vi "Micron Optics sm130 Triggered Acquisition.vi"() -> ()   [LabVIEW 2024]
doc: "Demonstrates the triggered peak wavelength acquisition. The peak wavelength acquisition can be untriggered, software or hardware triggered. \n\n<b>Note:</b>\nThis example is made for the instrument without channel multiplexer. Modifications will have to be made for instruments with channel multiplexer."
uses:
  Micron Optics sm130.lvlib
panel:
  in  "Trigger Type (0:Untriggered)":u16(ring) items=["Untriggered", "Software Triggered", "Hardware Triggered"]
  in  "Sensor Number (1)":i32=1
  in  "Channel (1: Channel 1)":i32(ring)=1 items=["Channel 1"=1, "Channel 2"=2, "Channel 3"=3, "Channel 4"=4]
  out "Peak Wavelength Chart":dbl(graph)
  in  "Stop":bool
  in  "Stop Trigger":bool
  in  "Start Trigger":bool
  in  "Data Interleave (1)":i32=1
  in  "Number of Acquisitions (100)":i32=100
  in  "Trigger Stop Condition (1:Edge Triggering)":u16(ring)=1 items=["Number of Acquisitions", "Edge Triggering"]
  in  "Trigger Stop Edge (0: Rising)":u16(ring) items=["Rising", "Falling"]
  in  "Trigger Start Edge (0: Rising)":u16(ring) items=["Rising", "Falling"]
  in  "VISA resource name":refnum<visa-resource-name>
  # "(c) 2009 - 2012 National Instruments.  ALL RIGHTS RESERVED."
  # "Sensor View"
  # "Trigger Control"
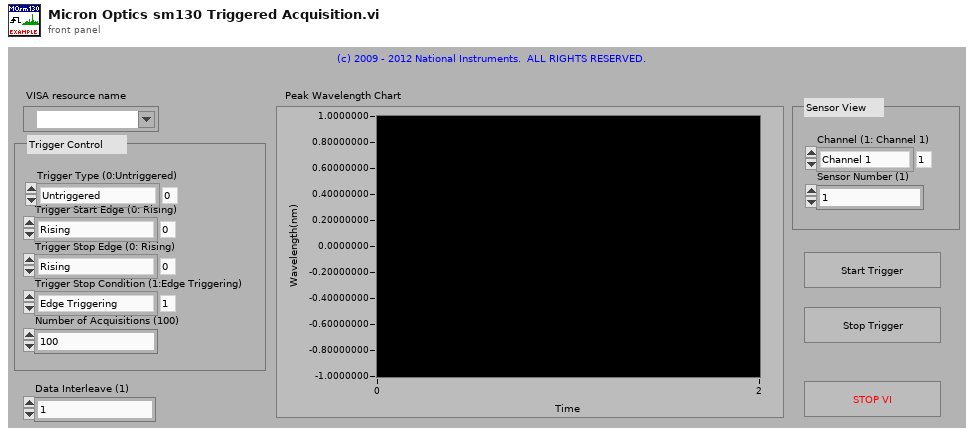
[diagram p1: front panel]
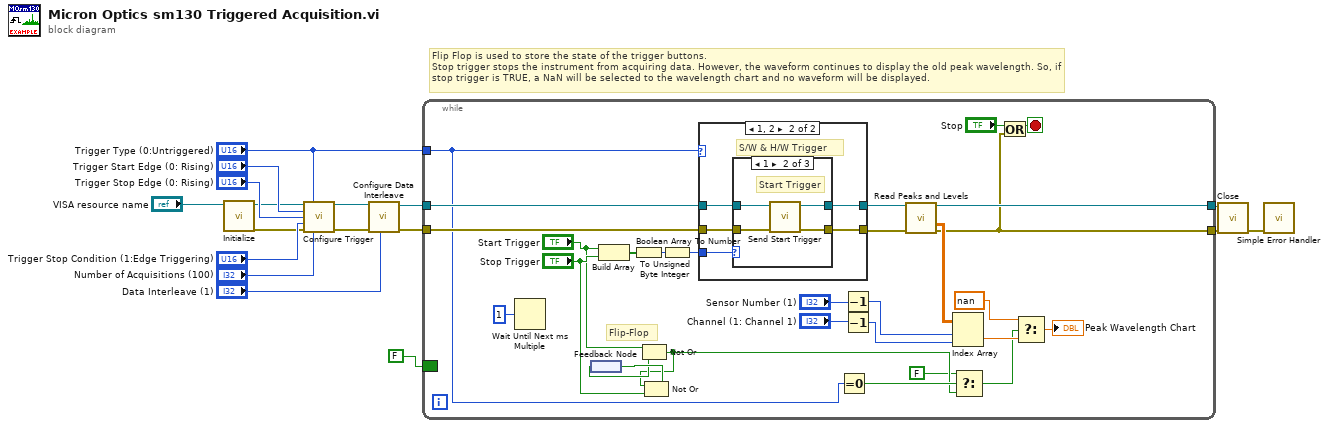
[diagram p0: block diagram]
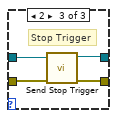
[diagram p4: hidden frame]
diagram:
  # "Flip Flop is used to store the state of the trigger buttons. \nStop trigger stops the instrument from acquiring data. However, the waveform continues to display the old peak wavelength. So, if stop trigger is TRUE, a NaN will be selected to the wavelength chart and no waveform will be displayed."
  n1 = call "Initialize.vi"("VISA resource name"="VISA resource name") -> ("error out"=w8:errorcluster, "VISA resource name out"=w9:refnum<visa-resource-name>)  [unwired: 9 in]
  n2 = call "Configure Trigger.vi"("VISA resource name"=w9, "Trigger Type (0:Untriggered)"="Trigger Type (0:Untriggered)", "Trigger Start Edge (0: Rising)"="Trigger Start Edge (0: Rising)", "Trigger Stop Edge (0: Rising)"="Trigger Stop Edge (0: Rising)", "Trigger Stop Condition (1:Edge Triggering)"="Trigger Stop Condition (1:Edge Triggering)", "error in (no error)"=w8, "Number of Acquisitions (100)"="Number of Acquisitions (100)") -> ("VISA resource name out"=w12:refnum<visa-resource-name>, "error out"=w11:errorcluster)  [unwired: 6 in, 1 out]
  n3 = call "Configure Data Interleave.vi"("Data Interleave (1)"="Data Interleave (1)", "error in (no error)"=w11, "VISA resource name"=w12) -> ("error out"=w5:errorcluster, "VISA resource name out"=w6:refnum<visa-resource-name>)  [unwired: 7 in]
  n4 = while {
    tunnel: w6 -> [w41]
    tunnel: w5 -> [w43]
    tunnel: "Trigger Type (0:Untriggered)" -> [w22]
    tunnel: [w26] -> w4
    tunnel: [w18] -> w3
    border: FALSE -> [_]
    stop <- w19 stop-if-true
    # "Flip-Flop"
    n5 = Wait Until Next ms Multiple(millisecond multiple=u32 1) -> ()  [unwired: 1 out]
    n6 = feedback #1() -> (w29:bool)
    n7 = Build Array("Start Trigger", "Stop Trigger") -> (w46:bool[])
    n8 = Boolean Array To Number(Boolean array=w46) -> (number=w45:u32)
    n9 = Not Or(1:w29, 2:"Start Trigger") -> (0:w23:bool)
    n10 = Not Or(1:"Stop Trigger", 2:w23) -> (0:w30:bool)
    n11 = feedback-in #1(w30) -> ()
    n12 = To Unsigned Byte Integer(number=w45) -> (unsigned 8bit integer=w44:u8)
    n13 = case shown="1, 2" w22 {
      tunnel: w44 -> [_ w53]
      tunnel: w41 -> [w48 w52]
      tunnel: w43 -> [w47 w51]
      tunnel: [w47 w50] -> w38
      tunnel: [w48 w49] -> w39
      frame 0, Default {
        # "Untriggered"
      }
      frame 1, 2 {
        # "S/W & H/W Trigger"
        n14 = case shown="1" w53 {
          tunnel: w52 -> [w55 w59 w63]
          tunnel: w51 -> [w54 w58 w60]
          tunnel: [w55 w57 w62] -> w49
          tunnel: [w54 w56 w61] -> w50
          frame 0, Default {
            # "No Trigger"
          }
          frame 1 {
            # "Start Trigger"
            n15 = call "Send Start Trigger.vi"("error in (no error)"=w58, "VISA resource name"=w59) -> ("error out"=w56:errorcluster, "VISA resource name out"=w57:refnum<visa-resource-name>)  [unwired: 8 in]
          }
          frame 2 {
            # "Stop Trigger"
            n16 = call "Send Stop Trigger.vi"("error in (no error)"=w60, "VISA resource name"=w63) -> ("error out"=w61:errorcluster, "VISA resource name out"=w62:refnum<visa-resource-name>)  [unwired: 8 in]
          }
        }
      }
    }
    n17 = Equal To 0?(x=w22) -> (x = 0?=w24:bool)
    n18 = Decrement(x="Sensor Number (1)") -> (x-1=w34:i32)
    n19 = Decrement(x="Channel (1: Channel 1)") -> (x-1=w33:i32)
    n20 = call "Read Peaks and Levels.vi"("VISA resource name"=w39, "error in (no error)"=w38) -> ("VISA resource name out"=w26:refnum<visa-resource-name>, "Peak Wavelengths (nm)"=w37:dbl[][], "error out"=w18:errorcluster)  [unwired: 5 in, 6 out]
    n21 = Index Array(array=w37, index (row)=w34, index (col)=w33) -> (element=w31:dbl)
    n22 = Select(t=FALSE, s=w24, f=w23) -> (s? t:f=w25:bool)
    n23 = Or(x="Stop", y=w18) -> (x .or. y?=w19:bool)
    n24 = Select(t=nan, s=w25, f=w31) -> (s? t:f=→"Peak Wavelength Chart":dbl)
  }
  n25 = call "Close.vi"("error in (no error)"=w3, "VISA resource name"=w4) -> ("error out"=w2:errorcluster)  [unwired: 9 in]
  n26 = call <vilib>:"Simple Error Handler.vi"("error in (no error)"=w2) -> ()  [unwired: 4 in, 5 out]
